vi "VectorNav Serial Port.vi"   [LabVIEW 2009]
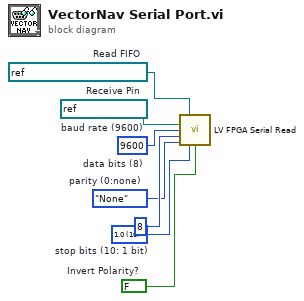
[diagram p0: block diagram]
diagram:
  w1 = FALSE  # Invert Polarity?
  w2 = u16 10 items=["1.0"=10, "1.5"=15, "2.0"=20]  # stop bits (10: 1 bit)
  w3 = enum16{"None", "Odd", "Even", "Mark", "Space"}."None"  # parity (0:none)
  w4 = 8  # data bits (8)
  w5 = u32 9600  # baud rate (9600)
  w6 = refnum<k21> "Port4/DIO3"  # Receive Pin
  w7 = refnum<k21> "VectorNav Read FIFO"  # Read FIFO
  n1 = call "LV FPGA Serial Read.vi"("Read FIFO"=w7, "Receive"=w6, "baud rate (9600)"=w5, "data bits (8)"=w4, "parity (0:none)"=w3, "stop bits (10: 1 bit)"=w2, "Invert Polarity?"=w1) -> ()  [unwired: 9 in]
